vi "工單號碼測試.vi"() -> ()   [LabVIEW 2019]
uses:
  Ctrl/Table Save.ctl
  LLB/Commonly VI/Main Glb.vi
  <vilib>/Utility/xml.llb/Write to XML File(string).vi
  <vilib>/Utility/xml.llb/Read From XML File(string).vi
  LLB/Commonly VI.lvlib
panel:
  in  "EnfMeasureTable 5":cluster{"Table Control":string[][]}[](array[cluster])
  out "工單號碼Table":cluster{"Table Control":string[][]}[](array[cluster])
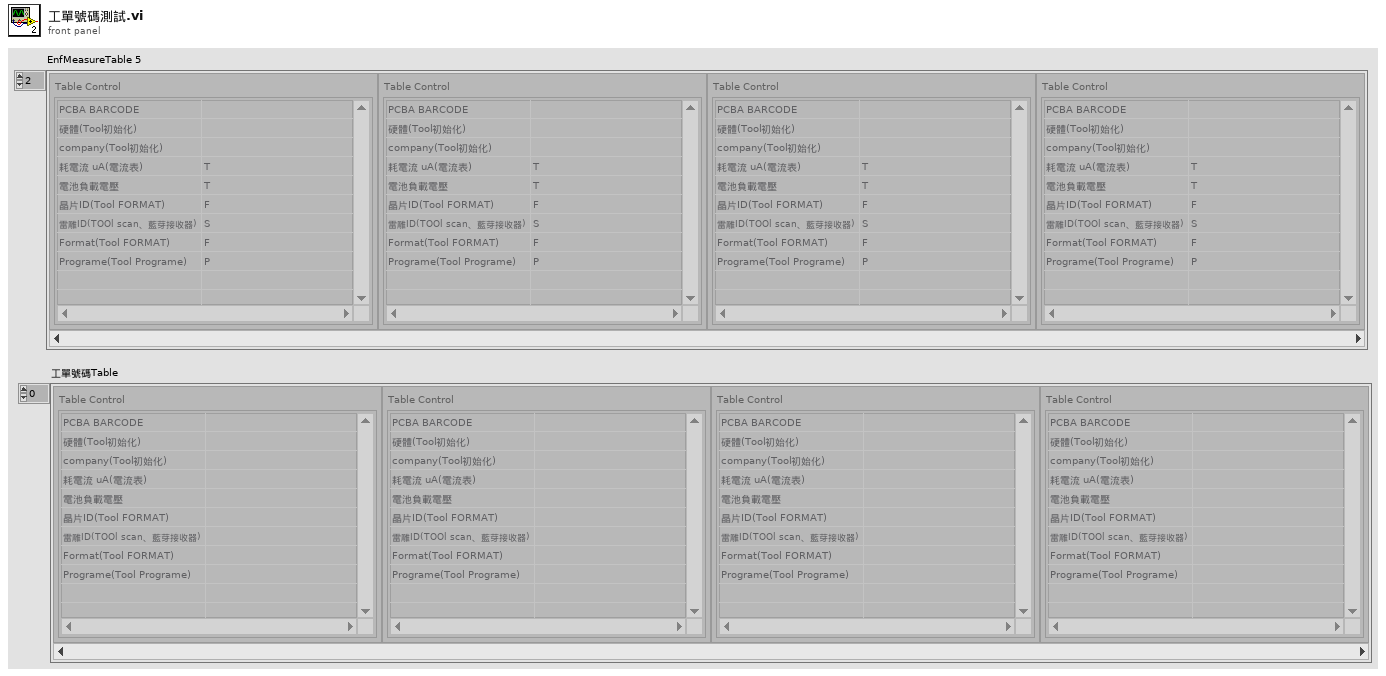
[diagram p1: front panel]
types:
  T1 = typedef "Table Save.ctl" = enum16{"initial", "Add", "Write", "Replace", "Delete", "REad", "RedTable", "Load"}
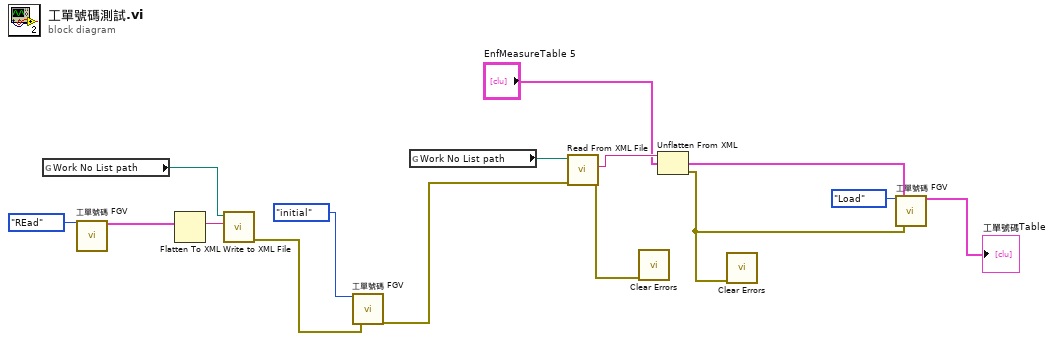
[diagram p0: block diagram]
diagram:
  n1 = global read "Main Glb.vi" "Work No List path"() -> (w15:path)
  n2 = call "工單號碼 FGV.vi"("Action"=Table_Save."REad") -> ("Total Table"=w13:cluster{"Table Control":string[][]}[])  [unwired: 11 in, 7 out]
  n3 = Flatten To XML(anything=w13) -> (xml string=w14:string)
  n4 = call-poly <vilib>:"Write to XML File.vi"("XML Input"=w14, "XML File Path"=w15) -> ("error out"=w3:errorcluster)  [unwired: 7 in, 2 out]
  n5 = call "工單號碼 FGV.vi"("Action"=Table_Save."initial", "error in (no error)"=w3) -> ("error out"=w2:errorcluster)  [unwired: 10 in, 7 out]
  n6 = global read "Main Glb.vi" "Work No List path"() -> (w11:path)
  n7 = call-poly <vilib>:"Read From XML File.vi"("error in (no error)"=w2, "XML File Path"=w11) -> ("error out"=w10:errorcluster, "XML Elements"=w9:string)  [unwired: 7 in, 1 out]
  n8 = call <vilib>:"Clear Errors.vi"("error in (no error)"=w10) -> ()  [unwired: 5 in, 2 out]
  n9 = Unflatten From XML(xml string=w9, type="EnfMeasureTable 5") -> (value=w1:cluster{"Table Control":string[][]}[], error out=w5:errorcluster)  [unwired: 1 in]
  n10 = call <vilib>:"Clear Errors.vi"("error in (no error)"=w5) -> ()  [unwired: 5 in, 2 out]
  n11 = call "工單號碼 FGV.vi"("Action"=Table_Save."Load", "Table Load"=w1, "error in (no error)"=w5) -> ("Total Table"=→"工單號碼Table":cluster{"Table Control":string[][]}[])  [unwired: 9 in, 7 out]
